vi "Read RS232.vi"() -> ()   [LabVIEW 2015]
uses:
  <vilib>/Instr/_visa.llb/Select Event Type.ctl
  <vilib>/Instr/_visa.llb/VISA Configure Serial Port (Instr).vi
  Global Data.vi
panel:
  out "error out":errorcluster
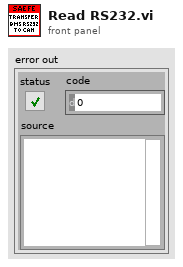
[diagram p1: front panel]
types:
  T1 = cluster{"read mode":enum16{"polling", "blocking"}, "write mode":enum16{"polling", "blocking"}}
  T2 = typedef "Select Event Type.ctl" = u32
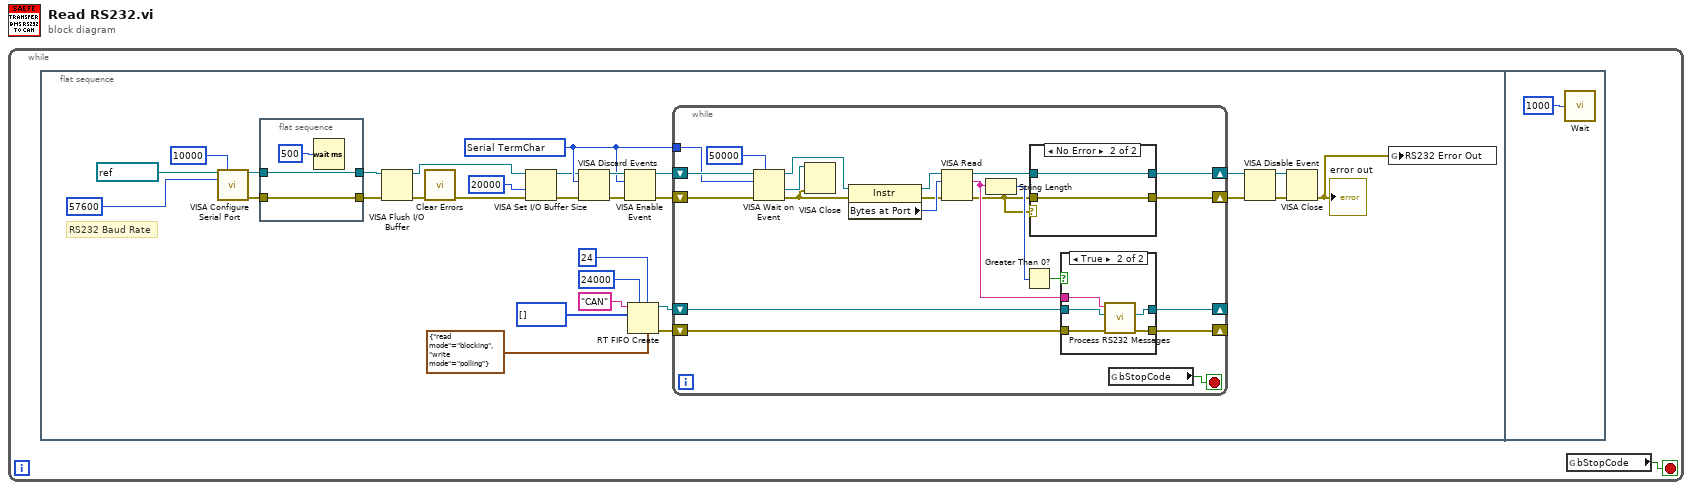
[diagram p0: block diagram]
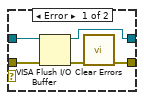
[diagram p2: hidden frame]
diagram:
  n1 = while {
    stop <- w1 stop-if-true
    n2 = flat-sequence {
      frame #0 {
        w11 = T2 1073684516 items=["Service Request"=1073684491, "Trigger"=3221168138, "Clear"=1073684493, "VXI Signal"=1073684512, "VXI/VME Interrupt"=3221168161, "VXI/VME Sysfail"=1073684509, "VXI/VME Sysreset"=1073684510, "GPIB CIC"=1073684498, "GPIB Talk"=1073684499, "GPIB Listen"=1073684500, "PXI Interrupt"=1073684514, "Serial Break"=1073684515, "Serial TermChar"=1073684516, "Serial CTS"=1073684521, "Serial DSR"=1073684522, "Serial DCD"=1073684524, "Serial RI"=1073684526, "Serial Character"=1073684533, "USB Interrupt"=1073684535, "All Enabled"=1073709055] ("Event Type")
        # "RS232 Baud Rate"
        n3 = call-poly "VISA Configure Serial Port"("VISA resource name"=refnum<visa-resource-name> "COM2", "timeout (10sec)"=u32 10000, "baud rate (9600)"=u32 57600 ("Baud Rate")) -> ("VISA resource name out"=w15:refnum<visa-resource-name>, "error out"=w14:errorcluster)  [unwired: 11 in]
        n4 = flat-sequence {
          tunnel: w15 -> [w34]
          tunnel: [w34] -> w9
          tunnel: w14 -> [w33]
          tunnel: [w33] -> w8
          frame #0 {
            n5 = Wait (ms)(milliseconds to wait=u32 500) -> ()  [unwired: 1 out]
          }
        }
        n6 = VISA Flush I/O Buffer(VISA resource name=w9, error in (no error)=w8) -> (VISA resource name out=w7:refnum<visa-resource-name>, error out=w6:errorcluster)  [unwired: 1 in]
        n7 = call <vilib>:"Clear Errors.vi"("error in (no error)"=w6) -> ("error out"=w5:errorcluster)  [unwired: 5 in, 1 out]
        n8 = VISA Set I/O Buffer Size(VISA resource name=w7, size (4096)=u32 20000, error in (no error)=w5) -> (VISA resource name out=w4:refnum<visa-resource-name>, error out=w3:errorcluster)  [unwired: 1 in]
        n9 = VISA Discard Events(8:w3, 10:w11, 11:w4) -> (0:w12:errorcluster, 3:w13:refnum<visa-resource-name>)  [unwired: 1 in]
        n10 = VISA Enable Event(8:w12, 10:w11, 11:w13) -> (0:w23:errorcluster, 3:w24:refnum<visa-resource-name>)  [unwired: 1 in]
        n11 = RT FIFO Create(0:"CAN" ("name (unnamed)"), 1:u8[] [], 4:u32 24000 ("size (10)"), 6:u32 24 ("elements in array (1)"), 7:T1 {"read mode"=enum."blocking", "write mode"=enum."polling"} ("r/w modes (polling,polling)")) -> (8:w26:refnum<k33>, 11:w25:errorcluster)  [unwired: 3 in, 1 out]
        n12 = while {
          shift-right: [w51] -> _
          shift-left: w26 -> [w53]
          shift-right: [w50] -> _
          shift-left: w25 -> [w52]
          shift-right: [w42] -> w18
          shift-left: w23 -> [w48]
          shift-right: [w43] -> w22
          shift-left: w24 -> [w49]
          tunnel: w11 -> [w46]
          stop <- w45 stop-if-true
          n13 = VISA Wait on Event(7:u32 50000 ("timeout (0)"), 8:w48, 10:w46, 11:w49) -> (0:w39:errorcluster, 1:w41:refnum<visa-resource-name>, 3:w40:refnum<visa-resource-name>)  [unwired: 1 in, 1 out]
          n14 = VISA Close(VISA resource name=w41, error in (no error)=w39) -> ()  [unwired: 1 out]
          n15 = property class="Instr"(reference=w40, error in=w39) -> (reference out=w37:refnum<visa-resource-name>, error out=w36:errorcluster, "Bytes at Port"=w38:u32)
          n16 = VISA Read(VISA resource name=w37, byte count=w38, error in (no error)=w36) -> (VISA resource name out=w44:refnum<visa-resource-name>, read buffer=w54:string, error out=w35:errorcluster)  [unwired: 1 out]
          n17 = String Length(string=w54) -> (length=w56:i32)
          n18 = Greater Than 0?(x=w56) -> (x > 0?=w55:bool)
          n19 = case shown="No Error" w35 {
            tunnel: w44 -> [w61 w63]
            tunnel: [w60 w63] -> w43
            tunnel: w35 -> [w59 w62]
            tunnel: [w57 w62] -> w42
            frame Error {
              n20 = VISA Flush I/O Buffer(VISA resource name=w61, error in (no error)=w59) -> (VISA resource name out=w60:refnum<visa-resource-name>, error out=w58:errorcluster)  [unwired: 1 in]
              n21 = call <vilib>:"Clear Errors.vi"("error in (no error)"=w58) -> ("error out"=w57:errorcluster)  [unwired: 5 in, 1 out]
            }
            frame No Error {
            }
          }
          n22 = case shown="True" w55 {
            tunnel: w54 -> [_ w70]
            tunnel: w53 -> [w65 w69]
            tunnel: w52 -> [w64 w68]
            tunnel: [w65 w67] -> w51
            tunnel: [w64 w66] -> w50
            frame False {
            }
            frame True {
              n23 = call "Process RS232 Messages.vi"("error in (no error)"=w68, "rt fifo"=w69, "BMS RS232 STRING"=w70) -> ("error out"=w66:errorcluster, "rt fifo out"=w67:refnum<k33>)  [unwired: 7 in]
            }
          }
          n24 = global read "Global Data.vi" "bStopCode"() -> (w45:bool)
        }
        n25 = VISA Disable Event(8:w18, 11:w22) -> (0:w20:errorcluster, 3:w21:refnum<visa-resource-name>)  [unwired: 2 in]
        n26 = VISA Close(VISA resource name=w21, error in (no error)=w20) -> (error out=w2:errorcluster)
        "error out" <- w2
        n27 = global write "Global Data.vi" "RS232 Error Out"(w2) -> ()
      }
      frame #1 {
        n28 = call "Wait"("Count(mSec)"=u32 1000) -> ()  [unwired: 1 out]
      }
    }
    n29 = global read "Global Data.vi" "bStopCode"() -> (w1:bool)
  }
